vi "Anritsu VNA Read Start and Stop Frequencies Boundaries.vi"(6 "Channel":i8=1 min=1 step=1, 7 "Anritsu VNA":T1, 8 "error in (no error)":errorcluster, 11 "VISA Resource Name":refnum<visa-resource-name>) -> (0 "error out":errorcluster, 2 "Start/Stop Freq Bounds, MHz":cluster{"Fstart":dbl, "Fstop":dbl}, 3 "dup VISA Resource Name":refnum<visa-resource-name>)   [LabVIEW 2011]
doc: "This VI for the HP8753B Network Analyzers reads the stimulus values. Except when performing log sweeps and freq list sweeps, this VI uses the start and stop values and the number of points to calcuate the stimulus values."
uses:
  TypeDefs/Anritsu VNA Instrument Info.ctl
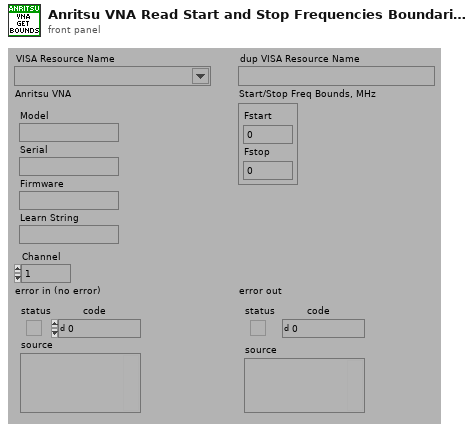
[diagram p1: front panel]
types:
  T1 = typedef "Anritsu VNA Instrument Info.ctl" = cluster{"Model":string, "Serial":string, "Firmware":string, "Learn String":string}
  T2 = typedef "Anritsu VNA Sweep Type.ctl" = enum32{"Linear Sweep", "Frequency Sweep", "Power Sweep", "CW Time Sweep", "Discrete Fill", "Time Domain", "Logarithmic Sweep", "Segmented Sweep (Frequency)", "Segmented Sweep (Index)", "MFGC"}
  T3 = typedef "Anritsu VNA Model.ctl" = enum16{"Not Supported", "37XXXX", "MS20XXX", "MS462XX", "MS464XX"}
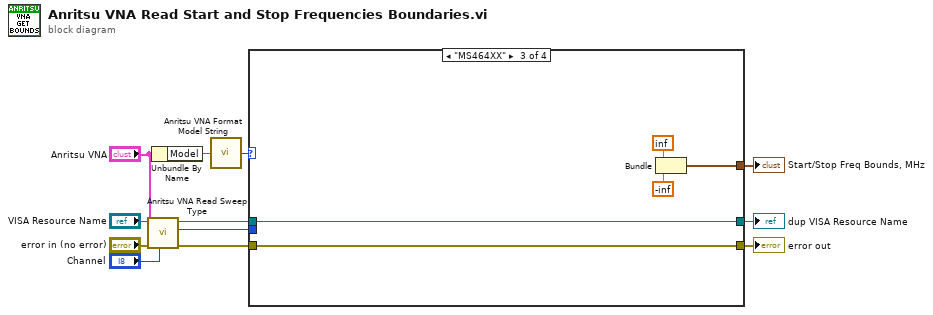
[diagram p0: block diagram]
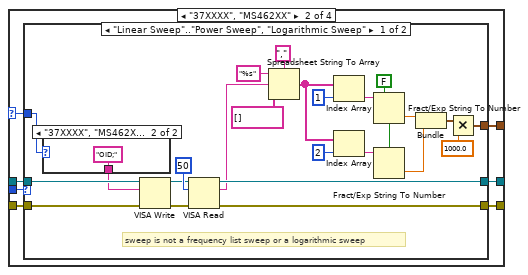
[diagram p3: hidden frame]
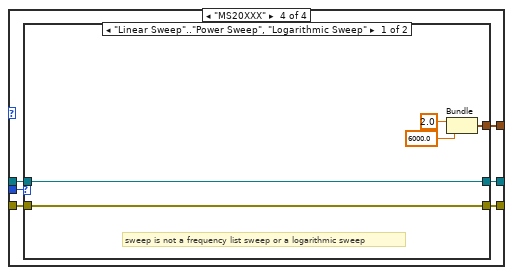
[diagram p6: hidden frame]
diagram:
  n1 = call "Anritsu VNA Read Sweep Type.vi"("Channel"="Channel", "Anritsu VNA"="Anritsu VNA", "error in (no error)"="error in (no error)", "VISA Resource Name"="VISA Resource Name") -> ("error out"=w7:errorcluster, "Sweep Type"=w10:T2, "dup VISA Resource Name"=w8:refnum<visa-resource-name>)  [unwired: 5 out]
  n2 = Unbundle By Name("Anritsu VNA") -> ("Model"=w3:string)
  n3 = call "Anritsu VNA Format Model String.vi"("Model"=w3) -> ("Model"=w2:T3)
  n4 = case shown="\"MS464XX\"" w2 {
    selector: w2 -> [_ w15 _ _]
    tunnel: [w13 w21 w49 w59] -> w12
    tunnel: w10 -> [_ w20 _ w58]
    tunnel: w8 -> [w14 w19 w50 w57]
    tunnel: w7 -> [w13 w18 w49 w56]
    tunnel: [_ w17 w53 w55] -> w6
    tunnel: [w14 w16 w50 w54] -> w5
    frame "Not Supported" {
    }
    frame "37XXXX", "MS462XX" {
      n5 = case shown="\"Linear Sweep\"..\"Power Sweep\", \"Logarithmic Sweep\"" w20 {
        tunnel: w19 -> [w42 w48]
        tunnel: w18 -> [w41 w47]
        tunnel: [w34 w47] -> w21
        tunnel: [w22 _] -> w17
        tunnel: [w35 w48] -> w16
        tunnel: w15 -> [w36 _]
        frame "Linear Sweep".."Power Sweep", "Logarithmic Sweep" {
          w23 = FALSE ("use system decimal point (T)")
          # "sweep is not a frequency list sweep or a logarithmic sweep"
          n6 = case shown="\"37XXXX\", \"MS462XX\"" w36 {
            tunnel: [_ "OID;"] -> w37
            frame "Not Supported", "MS20XXX", "MS464XX" {
            }
            frame "37XXXX", "MS462XX" {
            }
          }
          n7 = VISA Write(VISA resource name=w42, write buffer=w37, error in (no error)=w41) -> (VISA resource name out=w43:refnum<visa-resource-name>, error out=w45:errorcluster)  [unwired: 1 out]
          n8 = VISA Read(VISA resource name=w43, byte count=u32 50, error in (no error)=w45) -> (VISA resource name out=w35:refnum<visa-resource-name>, read buffer=w30:string, error out=w34:errorcluster)  [unwired: 1 out]
          n9 = Spreadsheet String To Array(delimiter (Tab)=",", format string="%s", spreadsheet string=w30, array type (2D Dbl)=string[] []) -> (array=w26:string[])
          n10 = Index Array(array=w26, index=1) -> (element=w25:string)
          n11 = Index Array(array=w26, index=2) -> (element=w24:string)
          n12 = Fract/Exp String To Number(use system decimal point (T)=w23, string=w25) -> (number=w39:dbl)  [unwired: 3 out]
          n13 = Fract/Exp String To Number(use system decimal point (T)=w23, string=w24) -> (number=w29:dbl)  [unwired: 3 out]
          n14 = Bundle(w39, w29) -> (w38:cluster{dbl, dbl})  [unwired: 1 out]
          n15 = Multiply(x=w38, y=1000.0) -> (x*y=w22:cluster{dbl, dbl})
        }
        frame "CW Time Sweep".."Time Domain", "Segmented Sweep (Frequency)".."MFGC" {
        }
      }
    }
    frame "MS464XX" {
      n16 = Bundle(inf, -inf) -> (w53:cluster{dbl, dbl})  [unwired: 1 out]
    }
    frame "MS20XXX" {
      n17 = case shown="\"Linear Sweep\"..\"Power Sweep\", \"Logarithmic Sweep\"" w58 {
        tunnel: w57 -> [w64 w66]
        tunnel: w56 -> [w63 w65]
        tunnel: [w63 w65] -> w59
        tunnel: [w60 _] -> w55
        tunnel: [w64 w66] -> w54
        frame "Linear Sweep".."Power Sweep", "Logarithmic Sweep" {
          # "sweep is not a frequency list sweep or a logarithmic sweep"
          n18 = Bundle(2.0, 6000.0) -> (w60:cluster{dbl, dbl})  [unwired: 1 out]
        }
        frame "CW Time Sweep".."Time Domain", "Segmented Sweep (Frequency)".."MFGC" {
        }
      }
    }
  }
  "dup VISA Resource Name" <- w5
  "error out" <- w12
  "Start/Stop Freq Bounds, MHz" <- w6
